vi "exec.vi"(8 "error in (no error)":errorcluster, 10 "context":refnum<class "Context.lvclass">, 11 "SwitchToOnDemandMode in":refnum<class "SwitchToOnDemandMode.lvclass">) -> (0 "error out":errorcluster, 2 "context 2":refnum<class "Context.lvclass">, 3 "SwitchToOnDemandMode out":refnum<class "SwitchToOnDemandMode.lvclass">)   [LabVIEW 2013, in "SwitchToOnDemandMode.lvclass"]
uses:
  SwitchToOnDemandMode.lvclass
  Context/Context.lvclass
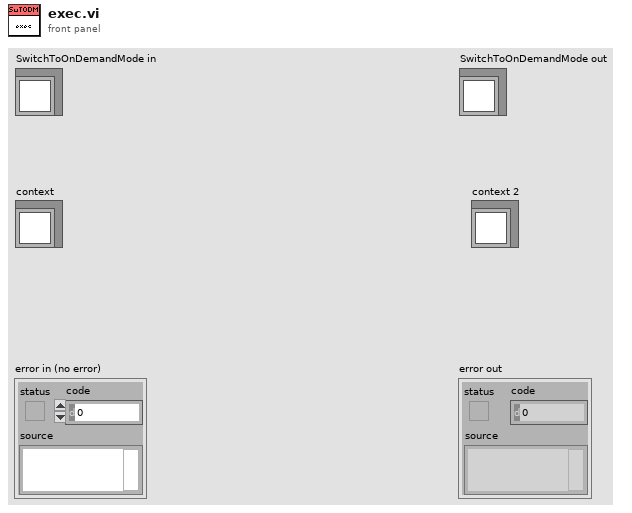
[diagram p1: front panel]
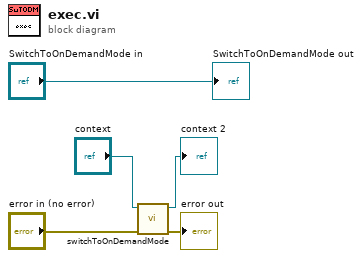
[diagram p0: block diagram]
diagram:
  n1 = call "switchToOnDemandMode.vi"("error in (no error)"="error in (no error)", "Context in"="context") -> ("error out"=→"error out":errorcluster, "Context out"=→"context 2":refnum<class "Context.lvclass">)  [unwired: 8 in]
  "SwitchToOnDemandMode out" <- "SwitchToOnDemandMode in"
